vi "Modulator.vi"(0 "input":T3={"signal"=[0.0, 0.0, 0.0, 0.0]}, 1 "modRegisters":T1={"numberOfInterleaves"="Register", "Enable"="Register", "triangleInc"="Register", "Deadband"="Register", "Enabled"="Register"}, 11 "Disable":bool) -> (4 "output":T2[](array[typedef]))   [LabVIEW 2017, in "BuckBoost.lvlib"]
uses:
  BuckBoost.lvlib
  modInput.ctl
  modOutput.ctl
  modRegisters.ctl
  modParameters.ctl
  <vilib>/Utility/error.llb/Clear Errors.vi
  <vilib>/rvi/Emulation/niFpgaSctlEmulationGetInTimedLoop.vi
  <vilib>/rvi/DataTransferAndStorage/Container/Common/niFpgaContainerExecOnDevCompGetState.vi
  <vilib>/rvi/Emulation/niFpgaEmulationIsFPGAContextNoSignature.vi
  <vilib>/rvi/DataTransferAndStorage/Container/Common/niFpgaContainerGetUniqueNameForEmu.vi
  <vilib>/rvi/Memory/Memory_Emulation/niFpgaMemoryEmulationCacheClearOnFirstRun.vi
  <vilib>/rvi/Memory/Memory_Emulation/nirvimemoryEmulationManagerCache_MakeExclusive.vi
  <vilib>/rvi/Memory/Memory_Emulation/niFpgaMemoryEmulationValidateCache.vi
  <vilib>/rvi/Memory/Memory_Emulation/nirvimemoryEmulationManagerCache_InsertValue.vi
  <vilib>/rvi/Memory/Memory_Emulation/nirvimemoryEmulationManagerCache_ReleaseExclusive.vi
  <vilib>/rvi/Memory/Memory_Emulation/nirvimemoryEmulationManagerCache_GetValue.vi
  <vilib>/rvi/Memory/Memory_Emulation/nirvimemoryEmulationManagerCache_SetValue.vi
  <vilib>/rvi/Emulation/niFpgaProcessEmulError.vi
  <vilib>/rvi/DataTransferAndStorage/Container/XNode/niFpgaContainer.xnode
  <vilib>/rvi/DataTransferAndStorage/Register/Emulation/niFpgaRegisterEmulationRefIn.vi
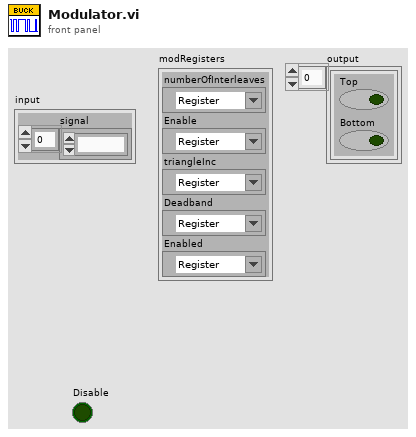
[diagram p1: front panel]
types:
  T1 = typedef "BuckBoost.lvlib/modRegisters.ctl" = cluster{"numberOfInterleaves":refnum<k21>, "Enable":refnum<k21>, "triangleInc":refnum<k21>, "Deadband":refnum<k21>, "Enabled":refnum<k21>}
  T2 = typedef "BuckBoost.lvlib/modOutput.ctl" = cluster{"Top":bool, "Bottom":bool}
  T3 = typedef "BuckBoost.lvlib/modInput.ctl" = cluster{"signal":fxp<+,18,0>[]}
  T4 = typedef "BuckBoost.lvlib/modParameters.ctl" = cluster{"triangleInc":fxp<+,18,0>, "Deadband":u16}
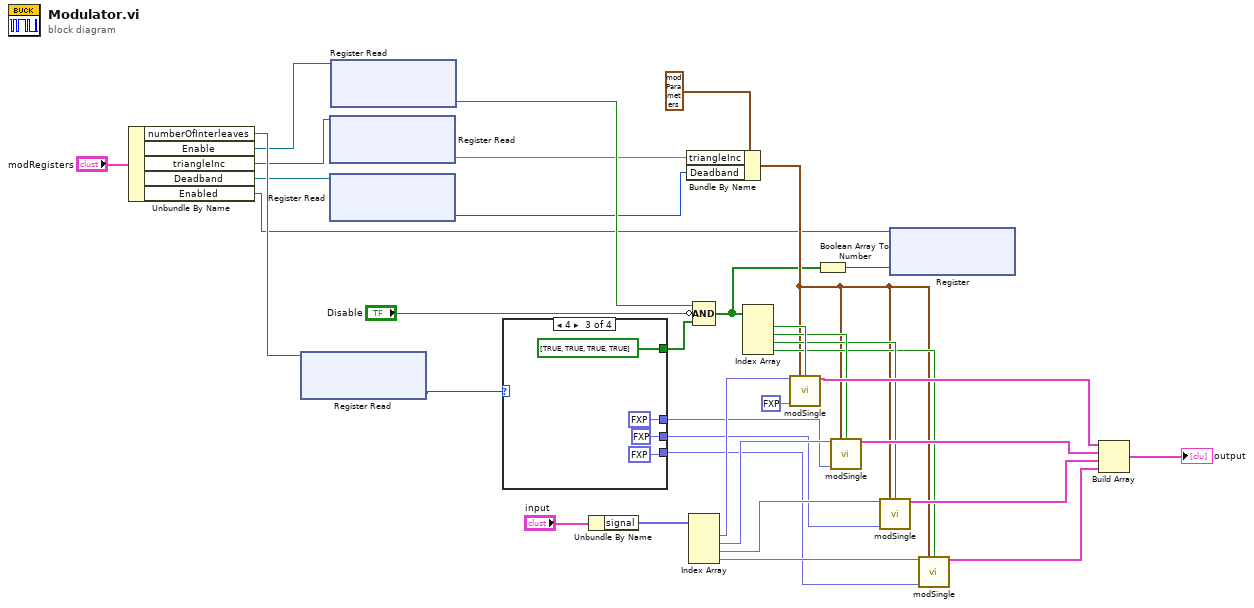
[diagram p0: block diagram]
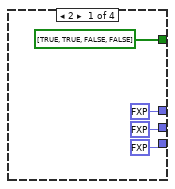
[diagram p2: hidden frame]
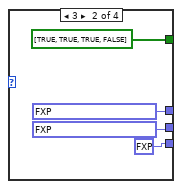
[diagram p3: hidden frame]
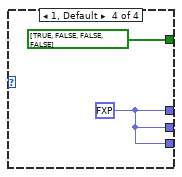
[diagram p4: hidden frame]
diagram:
  n1 = Unbundle By Name("modRegisters") -> ("numberOfInterleaves"=w13:refnum<k21>, "Enable"=w11:refnum<k21>, "triangleInc"=w9:refnum<k21>, "Deadband"=w6:refnum<k21>, "Enabled"=w1:refnum<k21>)
  n2 = xnode ("Register Read")("Register In"=w13) -> ("Data"=w12:u8)  [unwired: 1 out]
  n3 = xnode ("Register Read")("Register In"=w9) -> ("Data"=w7:fxp<+,18,0>)  [unwired: 1 out]
  n4 = xnode ("Register Read")("Register In"=w6) -> ("Data"=w5:u16)  [unwired: 1 out]
  n5 = xnode ("Register Read")("Register In"=w11) -> ("Data"=w10:bool)  [unwired: 1 out]
  n6 = case shown="4" w12 {
    tunnel: [bool[] [TRUE, TRUE, FALSE, FALSE] bool[] [TRUE, TRUE, TRUE, FALSE] bool[] [TRUE, TRUE, TRUE, TRUE] bool[] [TRUE, FALSE, FALSE, FALSE]] -> w23
    tunnel: [fxp<+,19,1> 1.0 ("triangleOffset") fxp<+,19,1> 0.6666679382324219 ("triangleOffset") fxp<+,19,1> 0.5 ("triangleOffset") w48] -> w18
    tunnel: [fxp<+,19,1> 0.0 ("triangleOffset") fxp<+,19,1> 1.3333320617675781 ("triangleOffset") fxp<+,19,1> 1.0 ("triangleOffset") w48] -> w17
    tunnel: [fxp<+,19,1> 0.0 ("triangleOffset") fxp<+,19,1> 0.0 ("triangleOffset") fxp<+,19,1> 1.5 ("triangleOffset") w48] -> w16
    frame 2 {
    }
    frame 3 {
    }
    frame 4 {
    }
    frame 1, Default {
      w48 = fxp<+,19,1> 0.0 ("triangleOffset")
    }
  }
  n7 = Unbundle By Name("input") -> ("signal"=w34:fxp<+,18,0>[])
  n8 = Bundle By Name(cluster=T4 {"triangleInc"=0.0, "Deadband"=0} ("Parameters"), "triangleInc"=w7, "Deadband"=w5) -> (w4:T4)
  n9 = Index Array(array=w34) -> (element #1=w33:fxp<+,18,0>, element #2=w32:fxp<+,18,0>, element #3=w31:fxp<+,18,0>, element #4=w30:fxp<+,18,0>)  [unwired: 4 in]
  n10 = Compound Arithmetic op=AND(w10, invert "Disable", w23) -> (w3:bool[])
  n11 = Index Array(array=w3) -> (element #1=w22:bool, element #2=w21:bool, element #3=w20:bool, element #4=w19:bool)  [unwired: 4 in]
  n12 = call "modSingle.vi"("signal"=w33, "Parameters"=w4, "Enable"=w22, "triangleOffset"=fxp<+,19,1> 0.0) -> ("output"=w29:T2)  [unwired: 11 in]
  n13 = Boolean Array To Number(Boolean array=w3) -> (number=w2:u8)
  n14 = call "modSingle.vi"("signal"=w32, "Parameters"=w4, "Enable"=w21, "triangleOffset"=w18) -> ("output"=w28:T2)  [unwired: 11 in]
  n15 = call "modSingle.vi"("signal"=w31, "Parameters"=w4, "Enable"=w20, "triangleOffset"=w17) -> ("output"=w27:T2)  [unwired: 11 in]
  n16 = xnode "Register"("Data"=w2, "Register In"=w1) -> ()  [unwired: 1 out]
  n17 = call "modSingle.vi"("signal"=w30, "Parameters"=w4, "Enable"=w19, "triangleOffset"=w16) -> ("output"=w26:T2)  [unwired: 11 in]
  n18 = Build Array(w29, w28, w27, w26) -> (→"output":T2[])
